vi "FeedbackDecode_Params2UEA.vi"(2 "StimClustIn":T1={"ParamsTable"=[], "Sel"=[], "Stim"=FALSE, "StimMode"=enum."Off", "StimStep"=[enum."1uA", enum."1uA", enum."Off"], "Jitter"=FALSE, "Pulse"=FALSE, "BFreq"=0.0, "BAmp"=0.0, "UEAArray"=[], "AdjClust"={"Add"=FALSE, "Sub"=FALSE, "Val"=[1.0, 100.0, 0.2, 500.0, 0.0], "B"=[FALSE, FALSE, FALSE, FALSE, FALSE], "Inc+"=["x+1", "x+10", "x+0.1", "x+10", "x+10"], "Set"=FALSE, "LoadTable"=FALSE, "SaveTable"=FALSE, "ClearTable"=FALSE, "DeleteSel"=FALSE, "Inc-"=["x-1", "x-10", "x-0.1", "x-10", "x-10"]}, "PresetTable"=[], "SelPreset"=[], "SortClust"={"Region"=FALSE, "Receptor"=FALSE, "Electrode"=FALSE, "Min Amp"=FALSE, "Max Amp"=FALSE, "Min Freq"=FALSE, "Max Freq"=FALSE, "Duration"=FALSE}, "SelSort"={"Sel"=FALSE}, "PresetClust"={"Load"=FALSE, "Clear"=FALSE, "Save"=FALSE, "Del"=FALSE}, "RespClust"={"RespType"=enum."Sensor Map", "OpenResp"=FALSE}, "AmpLimit"=0.0, "FreqLimit"=0.0, "DurLimit"=0.0, "Wait Period"=0.0, "Train Period"=0.0, "ManualType"=enum."Max"} {"Train Period" min=0.0 max=100.0 step=0.1; "Wait Period" min=0.0 max=100.0 step=0.1; "DurLimit" min=0.0 max=1.0 step=0.01; "FreqLimit" min=0.0 max=500.0 step=1.0; "AmpLimit" min=0.0 max=100.0 step=1.0; "BAmp" min=0.0 max=100.0 step=1.0; "BFreq" min=0.0 max=100.0 step=1.0}) -> (0 "StimClustOut":T1={"ParamsTable"=[], "Sel"=[], "Stim"=FALSE, "StimMode"=enum."Off", "StimStep"=[enum."1uA", enum."1uA", enum."Off"], "Jitter"=FALSE, "Pulse"=FALSE, "BFreq"=0.0, "BAmp"=0.0, "UEAArray"=[], "AdjClust"={"Add"=FALSE, "Sub"=FALSE, "Val"=[1.0, 100.0, 0.2, 500.0, 0.0], "B"=[FALSE, FALSE, FALSE, FALSE, FALSE], "Inc+"=["x+1", "x+10", "x+0.1", "x+10", "x+10"], "Set"=FALSE, "LoadTable"=FALSE, "SaveTable"=FALSE, "ClearTable"=FALSE, "DeleteSel"=FALSE, "Inc-"=["x-1", "x-10", "x-0.1", "x-10", "x-10"]}, "PresetTable"=[], "SelPreset"=[], "SortClust"={"Region"=FALSE, "Receptor"=FALSE, "Electrode"=FALSE, "Min Amp"=FALSE, "Max Amp"=FALSE, "Min Freq"=FALSE, "Max Freq"=FALSE, "Duration"=FALSE}, "SelSort"={"Sel"=FALSE}, "PresetClust"={"Load"=FALSE, "Clear"=FALSE, "Save"=FALSE, "Del"=FALSE}, "RespClust"={"RespType"=enum."Sensor Map", "OpenResp"=FALSE}, "AmpLimit"=0.0, "FreqLimit"=0.0, "DurLimit"=0.0, "Wait Period"=0.0, "Train Period"=0.0, "ManualType"=enum."Max"} {"Train Period" min=0.0 max=100.0 step=0.1; "Wait Period" min=0.0 max=100.0 step=0.1; "DurLimit" min=0.0 max=1.0 step=0.01; "FreqLimit" min=0.0 max=500.0 step=1.0; "AmpLimit" min=0.0 max=100.0 step=1.0; "BAmp" min=0.0 max=100.0 step=1.0; "BFreq" min=0.0 max=100.0 step=1.0})   [LabVIEW 2020]
uses:
  FeedbackDecode_EncodeClust.ctl
panel:
  # "Value"
  # "Inc-"
  # "Inc+"
  # "Min Amp"
  # "Max Amp"
  # "Min Freq"
  # "Max Freq"
  # "Duration"
  # "Value"
  # "Inc-"
  # "Inc+"
  # "Min Amp"
  # "Max Amp"
  # "Min Freq"
  # "Max Freq"
  # "Duration"
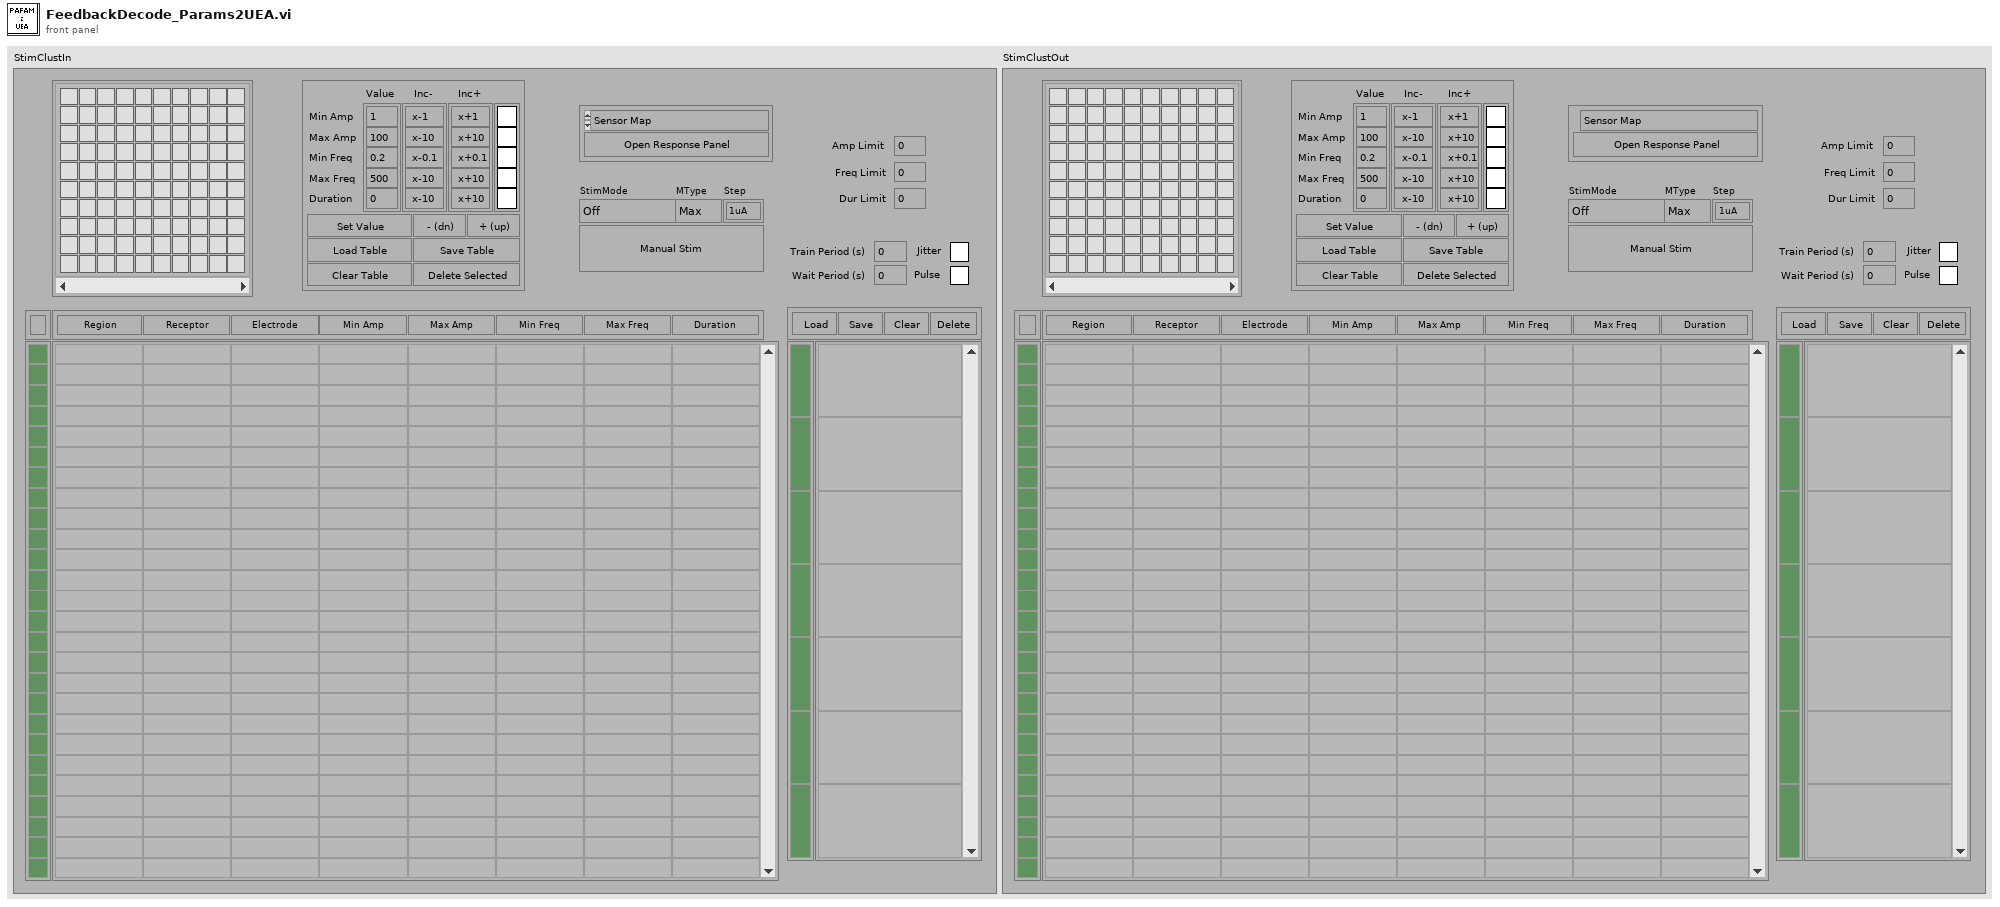
[diagram p1: front panel]
types:
  T1 = typedef "FeedbackDecode_EncodeClust.ctl" = cluster{"ParamsTable":string[][], "Sel":bool[], "Stim":bool, "StimMode":enum16{"Off", "Manual", "MSMS", "VRE", "3DHand", "DEKA", "Analog(DEKA)"}, "StimStep":enum16{"Off", "1uA", "2uA", "5uA", "10uA", "20uA", "30uA"}[], "Jitter":bool, "Pulse":bool, "BFreq":dbl, "BAmp":dbl, "UEAArray":cluster{"Boolean 1":bool, "Boolean 2":bool, "Boolean 3":bool, "Boolean 4":bool, "Boolean 5":bool, "Boolean 6":bool, "Boolean 7":bool, "Boolean 8":bool, "Boolean 9":bool, "Boolean 10":bool, "Boolean 11":bool, "Boolean 12":bool, "Boolean 13":bool, "Boolean 14":bool, "Boolean 15":bool, "Boolean 16":bool, "Boolean 17":bool, "Boolean 18":bool, "Boolean 19":bool, "Boolean 20":bool, "Boolean 21":bool, "Boolean 22":bool, "Boolean 23":bool, "Boolean 24":bool, "Boolean 25":bool, "Boolean 26":bool, "Boolean 27":bool, "Boolean 28":bool, "Boolean 29":bool, "Boolean 30":bool, "Boolean 31":bool, "Boolean 32":bool, "Boolean 33":bool, "Boolean 34":bool, "Boolean 35":bool, "Boolean 36":bool, "Boolean 37":bool, "Boolean 38":bool, "Boolean 39":bool, "Boolean 40":bool, "Boolean 41":bool, "Boolean 42":bool, "Boolean 43":bool, "Boolean 44":bool, "Boolean 45":bool, "Boolean 46":bool, "Boolean 47":bool, "Boolean 48":bool, "Boolean 49":bool, "Boolean 50":bool, "Boolean 51":bool, "Boolean 52":bool, "Boolean 53":bool, "Boolean 54":bool, "Boolean 55":bool, "Boolean 56":bool, "Boolean 57":bool, "Boolean 58":bool, "Boolean 59":bool, "Boolean 60":bool, "Boolean 61":bool, "Boolean 62":bool, "Boolean 63":bool, "Boolean 64":bool, "Boolean 65":bool, "Boolean 66":bool, "Boolean 67":bool, "Boolean 68":bool, "Boolean 69":bool, "Boolean 70":bool, "Boolean 71":bool, "Boolean 72":bool, "Boolean 73":bool, "Boolean 74":bool, "Boolean 75":bool, "Boolean 76":bool, "Boolean 77":bool, "Boolean 78":bool, "Boolean 79":bool, "Boolean 80":bool, "Boolean 81":bool, "Boolean 82":bool, "Boolean 83":bool, "Boolean 84":bool, "Boolean 85":bool, "Boolean 86":bool, "Boolean 87":bool, "Boolean 88":bool, "Boolean 89":bool, "Boolean 90":bool, "Boolean 91":bool, "Boolean 92":bool, "Boolean 93":bool, "Boolean 94":bool, "Boolean 95":bool, "Boolean 96":bool, "Boolean 97":bool, "Boolean 98":bool, "Boolean 99":bool, "Boolean 100":bool}[], "AdjClust":cluster{"Add":bool, "Sub":bool, "Val":dbl[], "B":bool[], "Inc+":string[], "Set":bool, "LoadTable":bool, "SaveTable":bool, "ClearTable":bool, "DeleteSel":bool, "Inc-":string[]}, "PresetTable":string[][], "SelPreset":bool[], "SortClust":cluster{"Region":bool, "Receptor":bool, "Electrode":bool, "Min Amp":bool, "Max Amp":bool, "Min Freq":bool, "Max Freq":bool, "Duration":bool}, "SelSort":cluster{"Sel":bool}, "PresetClust":cluster{"Load":bool, "Clear":bool, "Save":bool, "Del":bool}, "RespClust":cluster{"RespType":enum16{"Sensor Map", "Full Map"}, "OpenResp":bool}, "AmpLimit":dbl, "FreqLimit":dbl, "DurLimit":dbl, "Wait Period":dbl, "Train Period":dbl, "ManualType":enum16{"Max", "Min"}}
  T2 = cluster{"[0]":bool, "[1]":bool, "[2]":bool, "[3]":bool, "[4]":bool, "[5]":bool, "[6]":bool, "[7]":bool, "[8]":bool, "[9]":bool, "[10]":bool, "[11]":bool, "[12]":bool, "[13]":bool, "[14]":bool, "[15]":bool, "[16]":bool, "[17]":bool, "[18]":bool, "[19]":bool, "[20]":bool, "[21]":bool, "[22]":bool, "[23]":bool, "[24]":bool, "[25]":bool, "[26]":bool, "[27]":bool, "[28]":bool, "[29]":bool, "[30]":bool, "[31]":bool, "[32]":bool, "[33]":bool, "[34]":bool, "[35]":bool, "[36]":bool, "[37]":bool, "[38]":bool, "[39]":bool, "[40]":bool, "[41]":bool, "[42]":bool, "[43]":bool, "[44]":bool, "[45]":bool, "[46]":bool, "[47]":bool, "[48]":bool, "[49]":bool, "[50]":bool, "[51]":bool, "[52]":bool, "[53]":bool, "[54]":bool, "[55]":bool, "[56]":bool, "[57]":bool, "[58]":bool, "[59]":bool, "[60]":bool, "[61]":bool, "[62]":bool, "[63]":bool, "[64]":bool, "[65]":bool, "[66]":bool, "[67]":bool, "[68]":bool, "[69]":bool, "[70]":bool, "[71]":bool, "[72]":bool, "[73]":bool, "[74]":bool, "[75]":bool, "[76]":bool, "[77]":bool, "[78]":bool, "[79]":bool, "[80]":bool, "[81]":bool, "[82]":bool, "[83]":bool, "[84]":bool, "[85]":bool, "[86]":bool, "[87]":bool, "[88]":bool, "[89]":bool, "[90]":bool, "[91]":bool, "[92]":bool, "[93]":bool, "[94]":bool, "[95]":bool, "[96]":bool, "[97]":bool, "[98]":bool, "[99]":bool}
  T3 = cluster{"[0]":bool, "[1]":bool, "[2]":bool, "[3]":bool, "[4]":bool, "[5]":bool, "[6]":bool, "[7]":bool, "[8]":bool, "[9]":bool, "[10]":bool, "[11]":bool, "[12]":bool, "[13]":bool, "[14]":bool, "[15]":bool, "[16]":bool, "[17]":bool, "[18]":bool, "[19]":bool, "[20]":bool, "[21]":bool, "[22]":bool, "[23]":bool, "[24]":bool, "[25]":bool, "[26]":bool, "[27]":bool, "[28]":bool, "[29]":bool, "[30]":bool, "[31]":bool, "[32]":bool, "[33]":bool, "[34]":bool, "[35]":bool, "[36]":bool, "[37]":bool, "[38]":bool, "[39]":bool, "[40]":bool, "[41]":bool, "[42]":bool, "[43]":bool, "[44]":bool, "[45]":bool, "[46]":bool, "[47]":bool, "[48]":bool, "[49]":bool, "[50]":bool, "[51]":bool, "[52]":bool, "[53]":bool, "[54]":bool, "[55]":bool, "[56]":bool, "[57]":bool, "[58]":bool, "[59]":bool, "[60]":bool, "[61]":bool, "[62]":bool, "[63]":bool, "[64]":bool, "[65]":bool, "[66]":bool, "[67]":bool, "[68]":bool, "[69]":bool, "[70]":bool, "[71]":bool, "[72]":bool, "[73]":bool, "[74]":bool, "[75]":bool, "[76]":bool, "[77]":bool, "[78]":bool, "[79]":bool, "[80]":bool, "[81]":bool, "[82]":bool, "[83]":bool, "[84]":bool, "[85]":bool, "[86]":bool, "[87]":bool, "[88]":bool, "[89]":bool, "[90]":bool, "[91]":bool, "[92]":bool, "[93]":bool, "[94]":bool, "[95]":bool, "[96]":bool, "[97]":bool, "[98]":bool, "[99]":bool}[]
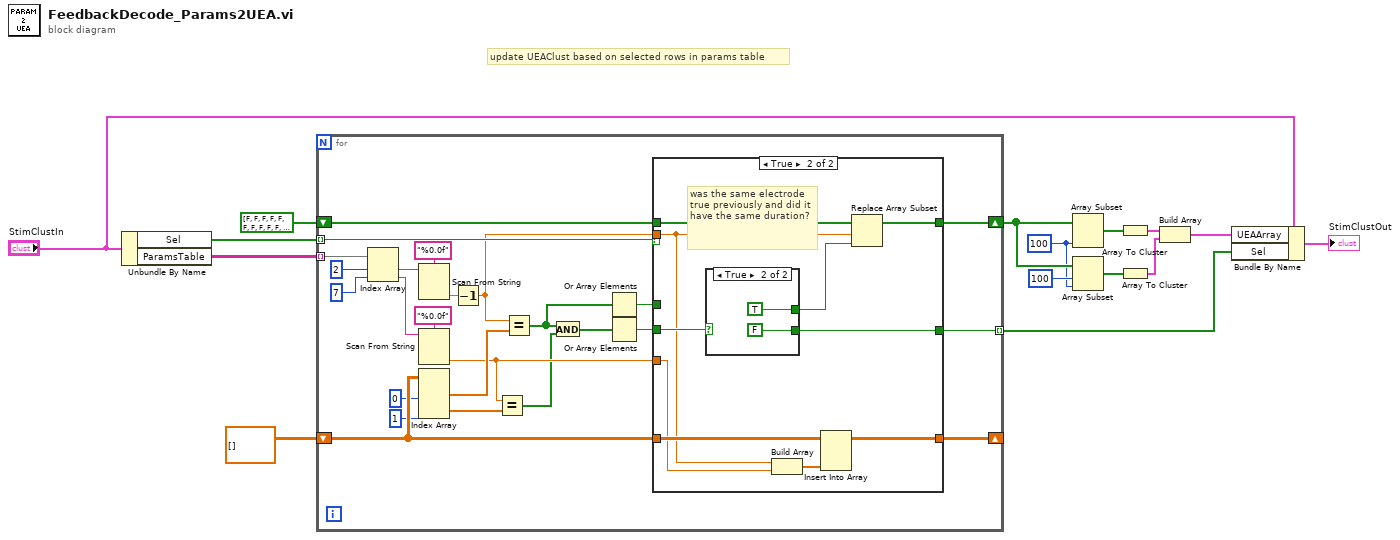
[diagram p0: block diagram]
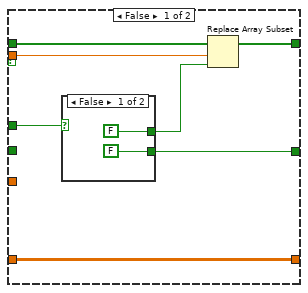
[diagram p2: hidden frame]
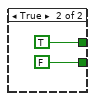
[diagram p3: hidden frame]
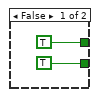
[diagram p4: hidden frame]
diagram:
  w6 = 100 ("length")
  # "update UEAClust based on selected rows in params table"
  n1 = Unbundle By Name("StimClustIn") -> ("Sel"=w11:bool[], "ParamsTable"=w10:string[][])
  n2 = for {
    tunnel: w11 -> [w34] mode=indexing
    tunnel: w10 -> [w40] mode=indexing
    shift-right: [w35] -> w8
    shift-left: bool[] [FALSE, FALSE, FALSE, FALSE, FALSE, FALSE, FALSE, FALSE, FALSE, FALSE, FALSE, FALSE, FALSE, FALSE, FALSE, FALSE, FALSE, FALSE, FALSE, FALSE, FALSE, FALSE, FALSE, FALSE, FALSE, FALSE, FALSE, FALSE, FALSE, FALSE, FALSE, FALSE, FALSE, FALSE, FALSE, FALSE, FALSE, FALSE, FALSE, FALSE, FALSE, FALSE, FALSE, FALSE, FALSE, FALSE, FALSE, FALSE, FALSE, FALSE, FALSE, FALSE, FALSE, FALSE, FALSE, FALSE, FALSE, FALSE, FALSE, FALSE, FALSE, FALSE, FALSE, FALSE, FALSE, FALSE, FALSE, FALSE, FALSE, FALSE, FALSE, FALSE, FALSE, FALSE, FALSE, FALSE, FALSE, FALSE, FALSE, FALSE, FALSE, FALSE, FALSE, FALSE, FALSE, FALSE, FALSE, FALSE, FALSE, FALSE, FALSE, FALSE, FALSE, FALSE, FALSE, FALSE, FALSE, FALSE, FALSE, FALSE, FALSE, FALSE, FALSE, FALSE, FALSE, FALSE, FALSE, FALSE, FALSE, FALSE, FALSE, FALSE, FALSE, FALSE, FALSE, FALSE, FALSE, FALSE, FALSE, FALSE, FALSE, FALSE, FALSE, FALSE, FALSE, FALSE, FALSE, FALSE, FALSE, FALSE, FALSE, FALSE, FALSE, FALSE, FALSE, FALSE, FALSE, FALSE, FALSE, FALSE, FALSE, FALSE, FALSE, FALSE, FALSE, FALSE, FALSE, FALSE, FALSE, FALSE, FALSE, FALSE, FALSE, FALSE, FALSE, FALSE, FALSE, FALSE, FALSE, FALSE, FALSE, FALSE, FALSE, FALSE, FALSE, FALSE, FALSE, FALSE, FALSE, FALSE, FALSE, FALSE, FALSE, FALSE, FALSE, FALSE, FALSE, FALSE, FALSE, FALSE, FALSE, FALSE, FALSE, FALSE, FALSE, FALSE, FALSE, FALSE, FALSE, FALSE, FALSE, FALSE, FALSE, FALSE, FALSE, FALSE, FALSE, FALSE, FALSE, FALSE] ("array") -> [w37]
    shift-right: [w33] -> _
    shift-left: dbl[][] [] -> [w26]
    tunnel: [w30] -> w12 mode=indexing
    n3 = Index Array(array=w40, index #1=2 ("index"), index #2=7 ("index")) -> (element #1=w39:string, element #2=w27:string)
    n4 = Scan From String(format string="%0.0f", input string=w39) -> (output 1=w36:dbl)  [unwired: 3 in, 3 out]
    n5 = Scan From String(format string="%0.0f", input string=w27) -> (output 1=w21:dbl)  [unwired: 3 in, 3 out]
    n6 = Index Array(array=w26, index (col) #1=0 ("disabled index (col)"), index (col) #2=1 ("index (col)")) -> (element #1=w25:dbl[], element #2=w22:dbl[])  [unwired: 2 in]
    n7 = Decrement(x=w36) -> (x-1=w32:dbl)
    n8 = Equal?(x=w21, y=w22) -> (x = y?=w20:bool[])
    n9 = Equal?(x=w32, y=w25) -> (x = y?=w18:bool[])
    n10 = And(x=w18, y=w20) -> (x .and. y?=w19:bool[])
    n11 = Or Array Elements(Boolean array=w18) -> (logical OR=w17:bool)
    n12 = Or Array Elements(Boolean array=w19) -> (logical OR=w31:bool)
    n13 = case shown="True" w34 {
      tunnel: w37 -> [w46 w61]
      tunnel: w32 -> [w42 w54]
      tunnel: [w45 w60] -> w35
      tunnel: w26 -> [w47 w58]
      tunnel: [w47 w59] -> w33
      tunnel: w31 -> [_ w57]
      tunnel: [w44 w56] -> w30
      tunnel: w21 -> [_ w53]
      tunnel: w17 -> [w41 _]
      frame False {
        n14 = case shown="False" w41 {
          tunnel: [FALSE ("new element/subarray") FALSE ("new element/subarray")] -> w44
          tunnel: [FALSE ("new element/subarray") TRUE ("new element/subarray")] -> w43
          frame False {
          }
          frame True {
          }
        }
        n15 = Replace Array Subset(array=w46, new element=w43, index=w42) -> (w45:bool[])
      }
      frame True {
        # "was the same electrode true previously and did it have the same duration?"
        n16 = case shown="True" w57 {
          tunnel: [TRUE ("new element/subarray") FALSE ("new element/subarray")] -> w56
          tunnel: [TRUE ("new element/subarray") TRUE ("new element/subarray")] -> w55
          frame False {
          }
          frame True {
          }
        }
        n17 = Build Array(w54, w53) -> (w52:dbl[])
        n18 = Insert Into Array(array=w58, new element=w52) -> (w59:dbl[][])  [unwired: 2 in]
        n19 = Replace Array Subset(array=w61, new element=w55, index=w54) -> (w60:bool[])
      }
    }
  }
  n20 = Array Subset(array=w8, length=w6) -> (w5:bool[])  [unwired: 1 in]
  n21 = Array Subset(array=w8, index=100 ("length"), length=w6) -> (w4:bool[])
  n22 = Array To Cluster(array=w5) -> (cluster=w3:T2)
  n23 = Array To Cluster(array=w4) -> (cluster=w2:T2)
  n24 = Build Array(w3, w2) -> (w1:T3)
  n25 = Bundle By Name(cluster="StimClustIn", "UEAArray"=w1, "Sel"=w12) -> (→"StimClustOut":T1)
